vi "_SetIsHubPort.vi"(8 "error in":errorcluster, 10 "IsHubPort":bool, 11 "Device In":u64) -> (0 "error out":errorcluster, 3 "Device Out":u64)   [LabVIEW 2012, in "Phidget Common.lvlib"]
uses:
  <instrlib>/Phidgets/Phidget Common/Phidget Common.lvlib
  phidget22.dll
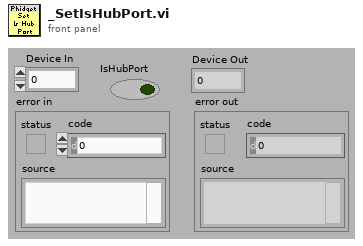
[diagram p1: front panel]
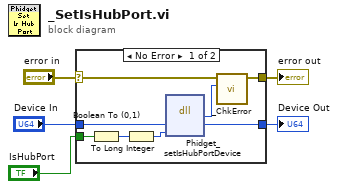
[diagram p0: block diagram]
diagram:
  n1 = case shown="No Error" "error in" {
    selector: "error in" -> [w11 w15]
    tunnel: [w9 w15] -> w4
    tunnel: "Device In" -> [w13 w14]
    tunnel: [w12 w14] -> w2
    tunnel: "IsHubPort" -> [w8 _]
    frame No Error {
      n2 = Boolean To (0,1)(Boolean=w8) -> (0, 1=w6:i16)
      n3 = To Long Integer(number=w6) -> (32bit integer=w7:i32)
      n4 = dll-call lib="phidget22.dll" fn="Phidget_setIsHubPortDevice"("phid"=w13, "HubPort"=w7) -> ("return type"=w10:i32, "phid"=w12:u64)  [unwired: 4 in, 2 out]
      n5 = call <instrlib>:"_ChkError.vi"("Return Code"=w10, "error in (no error)"=w11) -> ("error out"=w9:errorcluster)  [unwired: 9 in]
    }
    frame Error {
    }
  }
  "error out" <- w4
  "Device Out" <- w2
